vi "GetRTDProperties.vi"(11 "channel properties":T2[](array[typedef])) -> (3 "tdms properties":T1[](array[typedef]))   [LabVIEW 2017, in "Tdms.lvlib"]
uses:
  <vilib>/addons/InsightCM/Utilities/Tdms/Tdms.lvlib
  <vilib>/addons/InsightCM/MessageBus/Base/controls/KeyValuePair.ctl
  <vilib>/addons/InsightCM/Utilities/Tdms/controls/Property.ctl
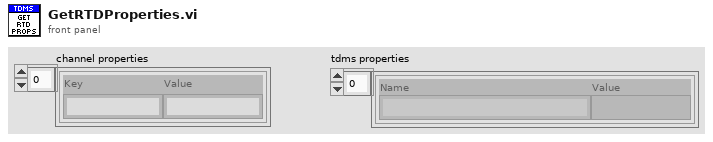
[diagram p1: front panel]
types:
  T1 = typedef "Tdms.lvlib/Property.ctl" = cluster{"Name":string, "Value":variant}
  T2 = typedef "KeyValuePair.ctl" = cluster{"Key":string, "Value":string}
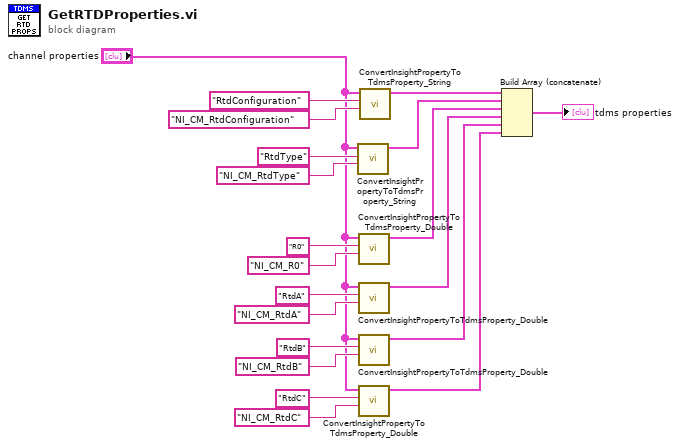
[diagram p0: block diagram]
diagram:
  n1 = call <vilib>:"ConvertInsightPropertyToTdmsProperty_String.vi"("Tdms Property Name"="NI_CM_RtdType" ("Name"), "Insight Property Name"="RtdType" ("Name"), "Insight Properties"="channel properties") -> ("Tdms Properties"=w8:T1[])  [unwired: 8 in]
  n2 = call <vilib>:"ConvertInsightPropertyToTdmsProperty_Double.vi"("Tdms Property Name"="NI_CM_R0" ("Name"), "Insight Property Name"="R0" ("Name"), "Insight Properties"="channel properties") -> ("Tdms Properties"=w16:T1[])  [unwired: 8 in]
  n3 = call <vilib>:"ConvertInsightPropertyToTdmsProperty_Double.vi"("Tdms Property Name"="NI_CM_RtdA" ("Name"), "Insight Property Name"="RtdA" ("Name"), "Insight Properties"="channel properties") -> ("Tdms Properties"=w15:T1[])  [unwired: 8 in]
  n4 = call <vilib>:"ConvertInsightPropertyToTdmsProperty_Double.vi"("Tdms Property Name"="NI_CM_RtdB" ("Name"), "Insight Property Name"="RtdB" ("Name"), "Insight Properties"="channel properties") -> ("Tdms Properties"=w2:T1[])  [unwired: 8 in]
  n5 = call <vilib>:"ConvertInsightPropertyToTdmsProperty_Double.vi"("Tdms Property Name"="NI_CM_RtdC" ("Name"), "Insight Property Name"="RtdC" ("Name"), "Insight Properties"="channel properties") -> ("Tdms Properties"=w1:T1[])  [unwired: 8 in]
  n6 = call <vilib>:"ConvertInsightPropertyToTdmsProperty_String.vi"("Tdms Property Name"="NI_CM_RtdConfiguration" ("Name"), "Insight Property Name"="RtdConfiguration" ("Name"), "Insight Properties"="channel properties") -> ("Tdms Properties"=w9:T1[])  [unwired: 8 in]
  n7 = Build Array (concatenate)(w9, w8, w16, w15, w2, w1) -> (→"tdms properties":T1[])
